vi "M686.vi"(4 "Special Function In":string, 6 "Velocity":dbl, 7 "Abort":refnum<vi>, 8 "Axis":bool[](array[boolean]), 9 "Positions":dbl[](array[numeric]), 10 "Action":T1=enum."MVR", 11 "VISA In":refnum<visa-resource-name>) -> (0 "Special Function Out":string, 1 "Status":bool, 2 "Position Out":dbl[](array[numeric]), 3 "VISA Out":refnum<visa-resource-name>)   [LabVIEW 2011]
uses:
  Controls/StageStates.ctl
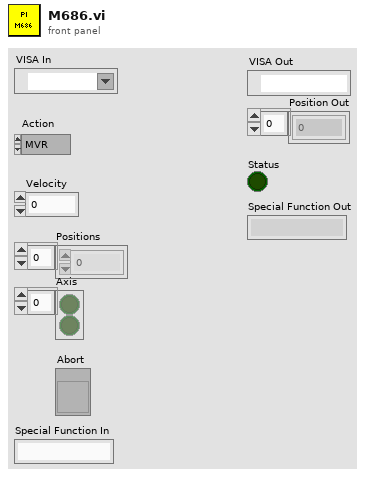
[diagram p1: front panel]
types:
  T1 = typedef "StageStates.ctl" = enum16{"POSITION", "MVR", "MOVE", "HALT", "ONTARGET", "ERROR", "EXIT", "HOME", "ZEROPOS", "NANOPOS", "QUIT", "ANALOG"}
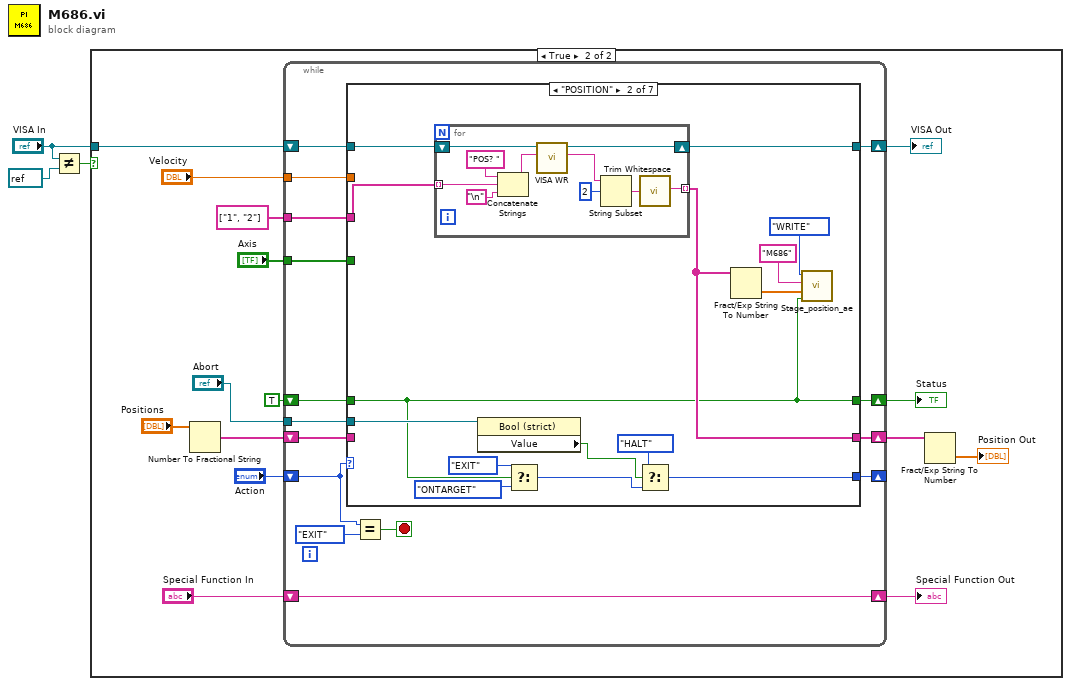
[diagram p0: block diagram]
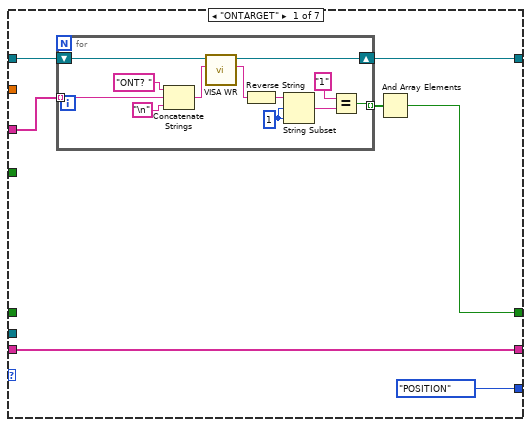
[diagram p3: hidden frame]
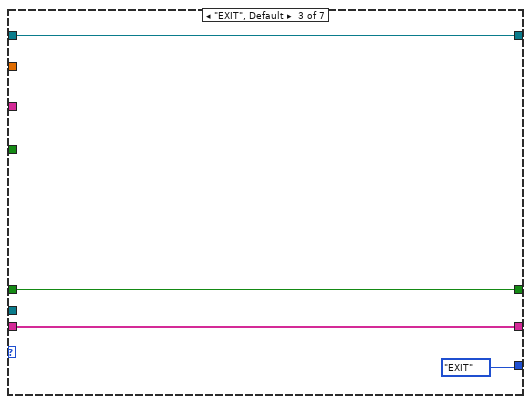
[diagram p4: hidden frame]
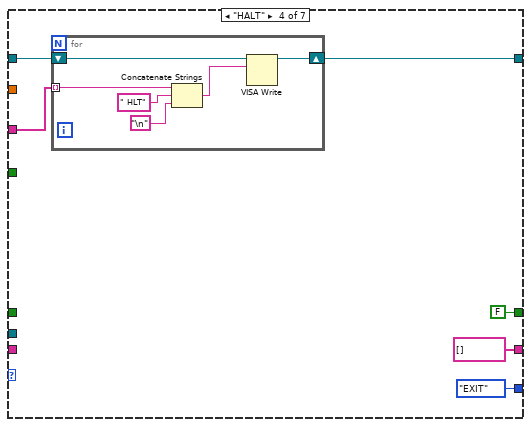
[diagram p5: hidden frame]
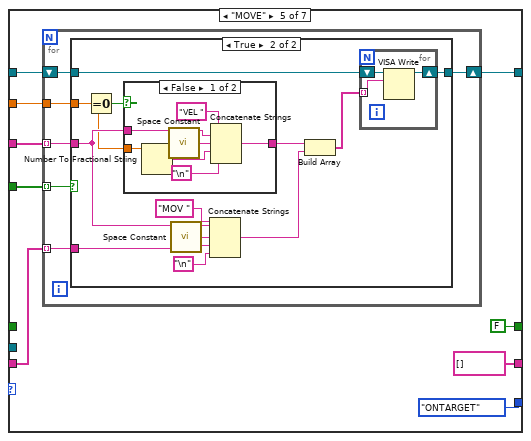
[diagram p6: hidden frame]
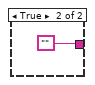
[diagram p8: hidden frame]
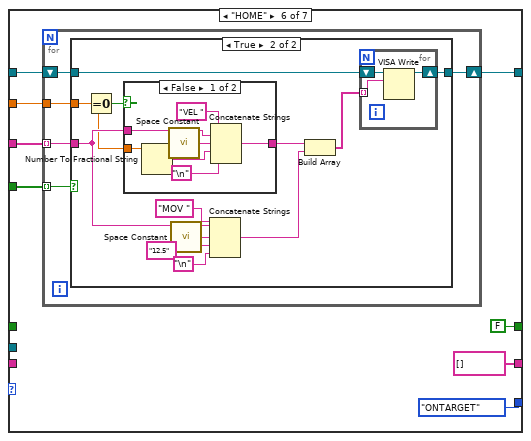
[diagram p9: hidden frame]
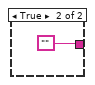
[diagram p11: hidden frame]
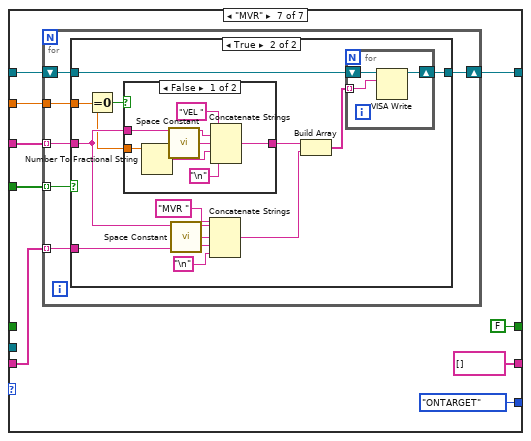
[diagram p12: hidden frame]
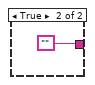
[diagram p14: hidden frame]
diagram:
  n1 = Not Equal?(x="VISA In", y=refnum<visa-resource-name> refnum ("VISA In")) -> (x != y?=w1:bool)
  n2 = case shown="True" w1 {
    tunnel: "VISA In" -> [_ w17]
    frame False {
    }
    frame True {
      n3 = Number To Fractional String(number="Positions") -> (F-format string=w10:string[])  [unwired: 3 in]
      n4 = while {
        tunnel: string[] ["1", "2"] -> [w33]
        shift-right: [w22] -> _
        shift-left: "Action" -> [w27]
        shift-right: [w30] -> w8
        shift-left: w10 -> [w31]
        shift-right: [w28] -> w15
        shift-left: TRUE -> [w29]
        tunnel: "Axis" -> [w26]
        tunnel: "Velocity" -> [w25]
        shift-right: [w24] -> w11
        shift-left: "Special Function In" -> [w24]
        shift-right: [w21] -> w5
        shift-left: w17 -> [w32]
        tunnel: "Abort" -> [w19]
        stop <- w20 stop-if-true
        n5 = case shown="\"POSITION\"" w27 {
          tunnel: w33 -> [w36 w66 _ w87 w102 w140 w178]
          tunnel: w32 -> [w40 w67 w78 w86 w101 w139 w177]
          tunnel: w31 -> [w38 _ w80 _ w100 _ w176]
          tunnel: [w38 w57 w80 string[] [] string[] [] string[] [] string[] []] -> w30
          tunnel: w29 -> [_ w53 w81 _ _ _ _]
          tunnel: [w37 w53 w81 FALSE FALSE FALSE FALSE] -> w28
          tunnel: w26 -> [_ _ _ _ w99 w138 w175]
          tunnel: w25 -> [_ _ _ _ w98 w137 w174]
          tunnel: [StageStates."POSITION" ("Action") w61 StageStates."EXIT" ("Action") StageStates."EXIT" ("Action") StageStates."ONTARGET" ("Action") StageStates."ONTARGET" ("Action") StageStates."ONTARGET" ("Action")] -> w22
          tunnel: [w34 w56 w78 w84 w96 w134 w172] -> w21
          tunnel: w19 -> [_ w55 _ _ _ _ _]
          frame "ONTARGET" {
            n6 = for {
              tunnel: [w47] -> w39 mode=indexing
              tunnel: w36 -> [w42] mode=indexing
              shift-right: [w41] -> w34
              shift-left: w40 -> [w52]
              w43 = 1 ("length (rest)")
              n7 = Concatenate Strings("ONT? " ("string"), w42, "\n") -> (w51:string)
              n8 = call "VISA WR.vi"("write buffer"=w51, "VISA Refnum in"=w52) -> ("read buffer"=w50:string, "VISA Refnum out"=w41:refnum<visa-resource-name>)  [unwired: 7 in, 1 out]
              n9 = Reverse String(1:w50) -> (0:w44:string)
              n10 = String Subset(string=w44, offset (0)=w43, length (rest)=w43) -> (substring=w49:string)
              n11 = Equal?(x="1", y=w49) -> (x = y?=w47:bool)
            }
            n12 = And Array Elements(Boolean array=w39) -> (logical AND=w37:bool)
          }
          frame "POSITION" {
            n13 = for {
              tunnel: [w74] -> w57 mode=indexing
              tunnel: w66 -> [w69] mode=indexing
              shift-right: [w68] -> w56
              shift-left: w67 -> [w77]
              n14 = Concatenate Strings("POS? " ("string"), w69, "\n") -> (w76:string)
              n15 = call "VISA WR.vi"("write buffer"=w76, "VISA Refnum in"=w77) -> ("read buffer"=w75:string, "VISA Refnum out"=w68:refnum<visa-resource-name>)  [unwired: 7 in, 1 out]
              n16 = String Subset(string=w75, offset (0)=2) -> (substring=w70:string)  [unwired: 1 in]
              n17 = call <vilib>:"Trim Whitespace.vi"("string"=w70) -> ("trimmed string"=w74:string)  [unwired: 1 in]
            }
            n18 = property class="Bool (strict)"(reference=w55) -> ("Value"=w54:bool)  [unwired: 1 in, 2 out]
            n19 = Select(t=StageStates."EXIT" ("Action"), s=w53, f=StageStates."ONTARGET" ("Action")) -> (s? t:f=w64:T1)
            n20 = Select(t=StageStates."HALT", s=w54, f=w64) -> (s? t:f=w61:T1)
            n21 = Fract/Exp String To Number(string=w57) -> (number=w58:dbl[])  [unwired: 3 in, 1 out]
            n22 = call "Stage_position_ae.vi"("Status In"=w53, "Position In"=w58, "StageID"="M686", "Enum"=enum16{"WRITE", "READ"}."WRITE") -> ()  [unwired: 6 in, 2 out]
          }
          frame "EXIT", Default {
          }
          frame "HALT" {
            n23 = for {
              tunnel: w87 -> [w91] mode=indexing
              shift-right: [w88] -> w84
              shift-left: w86 -> [w89]
              n24 = Concatenate Strings(w91, " HLT" ("string"), "\n") -> (w90:string)
              n25 = VISA Write(VISA resource name=w89, write buffer=w90) -> (VISA resource name out=w88:refnum<visa-resource-name>)  [unwired: 1 in, 2 out]
            }
          }
          frame "MOVE" {
            n26 = for {
              tunnel: w102 -> [w108] mode=indexing
              tunnel: w100 -> [w107] mode=indexing
              shift-right: [w105] -> w96
              shift-left: w101 -> [w106]
              tunnel: w99 -> [w104] mode=indexing
              tunnel: w98 -> [w103]
              n27 = case shown="True" w104 {
                tunnel: w108 -> [_ w115]
                tunnel: w107 -> [_ w118]
                tunnel: w106 -> [w109 w117]
                tunnel: [w109 w116] -> w105
                tunnel: w103 -> [_ w114]
                frame False {
                }
                frame True {
                  n28 = Equal To 0?(x=w114) -> (x = 0?=w113:bool)
                  n29 = case shown="False" w113 {
                    tunnel: w115 -> [w128 _]
                    tunnel: w114 -> [w125 _]
                    tunnel: [w127 ""] -> w112
                    frame False {
                      n30 = Number To Fractional String(number=w125) -> (F-format string=w126:string)  [unwired: 3 in]
                      n31 = call <vilib>:"Space Constant.vi"() -> ("String"=w131:string)
                      n32 = Concatenate Strings("VEL ", w128, w131, w126, "\n") -> (w127:string)
                    }
                    frame True {
                    }
                  }
                  n33 = call <vilib>:"Space Constant.vi"() -> ("String"=w119:string)
                  n34 = Concatenate Strings("MOV ", w115, w119, w118, "\n") -> (w111:string)
                  n35 = Build Array(w112, w111) -> (w110:string[])
                  n36 = for {
                    shift-right: [w123] -> w116
                    shift-left: w117 -> [w124]
                    tunnel: w110 -> [w122] mode=indexing
                    n37 = VISA Write(VISA resource name=w124, write buffer=w122) -> (VISA resource name out=w123:refnum<visa-resource-name>)  [unwired: 1 in, 2 out]
                  }
                }
              }
            }
          }
          frame "HOME" {
            n38 = for {
              tunnel: w140 -> [w145] mode=indexing
              shift-right: [w143] -> w134
              shift-left: w139 -> [w144]
              tunnel: w138 -> [w142] mode=indexing
              tunnel: w137 -> [w141]
              n39 = case shown="True" w142 {
                tunnel: w145 -> [_ w153]
                tunnel: w144 -> [w146 w155]
                tunnel: [w146 w154] -> w143
                tunnel: w141 -> [_ w152]
                frame False {
                }
                frame True {
                  n40 = Equal To 0?(x=w152) -> (x = 0?=w151:bool)
                  n41 = case shown="False" w151 {
                    tunnel: w153 -> [w165 _]
                    tunnel: w152 -> [w162 _]
                    tunnel: [w164 ""] -> w150
                    frame False {
                      n42 = Number To Fractional String(number=w162) -> (F-format string=w163:string)  [unwired: 3 in]
                      n43 = call <vilib>:"Space Constant.vi"() -> ("String"=w168:string)
                      n44 = Concatenate Strings("VEL ", w165, w168, w163, "\n") -> (w164:string)
                    }
                    frame True {
                    }
                  }
                  n45 = call <vilib>:"Space Constant.vi"() -> ("String"=w156:string)
                  n46 = Concatenate Strings("MOV ", w153, w156, "12.5" ("string"), "\n") -> (w149:string)
                  n47 = Build Array(w150, w149) -> (w148:string[])
                  n48 = for {
                    shift-right: [w160] -> w154
                    shift-left: w155 -> [w161]
                    tunnel: w148 -> [w159] mode=indexing
                    n49 = VISA Write(VISA resource name=w161, write buffer=w159) -> (VISA resource name out=w160:refnum<visa-resource-name>)  [unwired: 1 in, 2 out]
                  }
                }
              }
            }
          }
          frame "MVR" {
            n50 = for {
              tunnel: w178 -> [w184] mode=indexing
              tunnel: w176 -> [w183] mode=indexing
              shift-right: [w181] -> w172
              shift-left: w177 -> [w182]
              tunnel: w175 -> [w180] mode=indexing
              tunnel: w174 -> [w179]
              n51 = case shown="True" w180 {
                tunnel: w184 -> [_ w191]
                tunnel: w183 -> [_ w194]
                tunnel: w182 -> [w185 w193]
                tunnel: [w185 w192] -> w181
                tunnel: w179 -> [_ w190]
                frame False {
                }
                frame True {
                  n52 = Equal To 0?(x=w190) -> (x = 0?=w189:bool)
                  n53 = case shown="False" w189 {
                    tunnel: w191 -> [w204 _]
                    tunnel: w190 -> [w202 _]
                    tunnel: [w203 ""] -> w188
                    frame False {
                      n54 = Number To Fractional String(number=w202) -> (F-format string=w201:string)  [unwired: 3 in]
                      n55 = call <vilib>:"Space Constant.vi"() -> ("String"=w207:string)
                      n56 = Concatenate Strings("VEL ", w204, w207, w201, "\n") -> (w203:string)
                    }
                    frame True {
                    }
                  }
                  n57 = call <vilib>:"Space Constant.vi"() -> ("String"=w195:string)
                  n58 = Concatenate Strings("MVR ", w191, w195, w194, "\n") -> (w187:string)
                  n59 = Build Array(w188, w187) -> (w186:string[])
                  n60 = for {
                    shift-right: [w199] -> w192
                    shift-left: w193 -> [w200]
                    tunnel: w186 -> [w198] mode=indexing
                    n61 = VISA Write(VISA resource name=w200, write buffer=w198) -> (VISA resource name out=w199:refnum<visa-resource-name>)  [unwired: 1 in, 2 out]
                  }
                }
              }
            }
          }
        }
        n62 = Equal?(x=w27, y=StageStates."EXIT") -> (x = y?=w20:bool)
      }
      "Status" <- w15
      "Special Function Out" <- w11
      "VISA Out" <- w5
      n63 = Fract/Exp String To Number(string=w8) -> (number=→"Position Out":dbl[])  [unwired: 3 in, 1 out]
    }
  }
